vi "RedistributePathPoints.vi"(1 "Desired Point Spacing (in)":dbl, 2 "Path Length (in)":dbl, 3 "PathIn":T1[](array[typedef]), 4 "IndexedPathLength":dbl[](array[numeric])) -> (0 "PathOut":T1[](array[typedef]))   [LabVIEW 2017]
uses:
  TypeDefs/Point2D.ctl
  ArgosLib/ArgosLib.lvlib
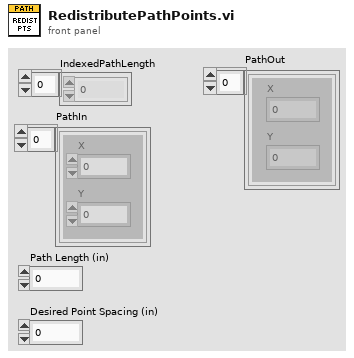
[diagram p1: front panel]
types:
  T1 = typedef "Point2D.ctl" = cluster{"X":dbl, "Y":dbl}
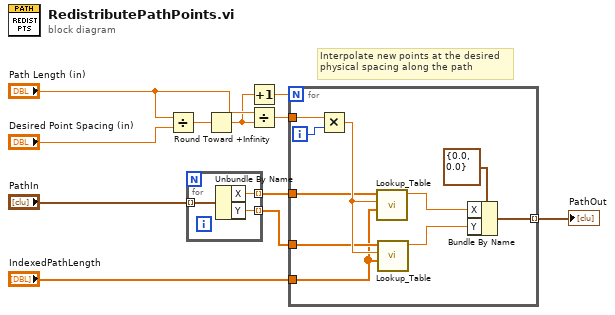
[diagram p0: block diagram]
diagram:
  # "Interpolate new points at the desired\nphysical spacing along the path"
  n1 = Divide(x="Path Length (in)", y="Desired Point Spacing (in)") -> (x/y=w10:dbl)
  n2 = for {
    tunnel: "PathIn" -> [w14] mode=indexing
    tunnel: [w13] -> w4 mode=indexing
    tunnel: [w12] -> w3 mode=indexing
    n3 = Unbundle By Name(w14) -> ("X"=w13:dbl, "Y"=w12:dbl)
  }
  n4 = Round Toward +Infinity(x=w10) -> (ceil(x): smallest int >= x=w6:dbl)
  n5 = Increment(x=w6) -> (x+1=w1:dbl)
  n6 = Divide(x="Path Length (in)", y=w6) -> (x/y=w8:dbl)
  n7 = for {
    N: w1 -> [_]
    tunnel: w8 -> [w23]
    tunnel: w4 -> [w21]
    tunnel: w3 -> [w20]
    tunnel: "IndexedPathLength" -> [w19]
    tunnel: [w15] -> w2 mode=indexing
    i -> [w24]
    n8 = Multiply(x=w23, y=w24) -> (x*y=w22:dbl)
    n9 = call "Lookup_Table.vi"("Y_Array"=w21, "x_in"=w22, "X_Array"=w19) -> ("y_out"=w17:dbl)  [unwired: 6 in]
    n10 = call "Lookup_Table.vi"("Y_Array"=w20, "x_in"=w22, "X_Array"=w19) -> ("y_out"=w16:dbl)  [unwired: 6 in]
    n11 = Bundle By Name(cluster=T1 {"X"=0.0, "Y"=0.0} ("2DPoint"), "X"=w17, "Y"=w16) -> (w15:T1)
  }
  "PathOut" <- w2
